vi "donut_fitting(subVI).vi"(5 "Edge Options":T1={"Edge Polarity"=0, "Kernel Size"=3, "Width"=3, "Minimum Edge Strength"=10.0, "Interpolation Type"=enum."Bilinear Fixed", "Data Processing Method"=enum."Average"} {"Edge Polarity" items=["All Edges", "Rising Edges", "Falling Edges"]; "Minimum Edge Strength" format="%.2f"; "Width" step=2; "Kernel Size" step=2}, 7 "Scan Direction":u16(ring) items=["Outside To Inside", "Inside To Outside"], 8 "error in (no error)":errorcluster, 9 "Step Size":dbl=5.0 format="%#_13g", 10 "image dest":T3, 11 "Image in":T3) -> (0 "error out":errorcluster, 3 "Image Out":T3)   [LabVIEW 2020]
uses:
  <vilib>/vision/Image Controls.llb/IMAQ Image.ctl
  <vilib>/vision/Measure.llb/Edge Options.ctl
  <vilib>/vision/Measure.llb/Edge Polarity.ctl
  <vilib>/vision/NI_Vision_Development_Module.lvlib
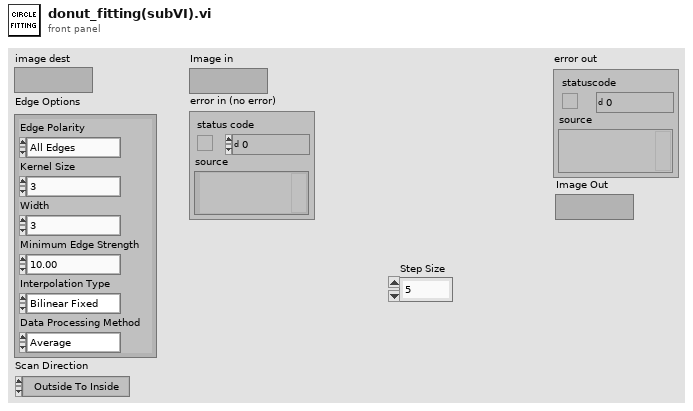
[diagram p1: front panel]
types:
  T1 = typedef "Edge Options.ctl" = cluster{"Edge Polarity":T2, "Kernel Size":u32, "Width":u32, "Minimum Edge Strength":sgl, "Interpolation Type":enum32{"Zero Order", "Bilinear", "Quadratic", "Cubic", "Bilinear Fixed"}, "Data Processing Method":enum32{"Average", "Median"}}
  T2 = typedef "Edge Polarity.ctl" = u32
  T3 = typedef "IMAQ Image.ctl" = refnum<image>
  T4 = typedef "ROI Descriptor" = cluster{"Global Rectangle":i32[], "Contours":cluster{"ID":enum32{"External", "Internal"}, "Type":u32, "Coordinates":i32[]}[]}
  T5 = typedef "Edge New.ctl" = cluster{"Location (Pixel)":cluster{"X":sgl, "Y":sgl}, "Location (Real-World)":cluster{"X":sgl, "Y":sgl}, "Distance (Pixel)":dbl, "Distance (Real-World)":dbl, "Strength":dbl, "Noise":dbl, "Rising?":bool}
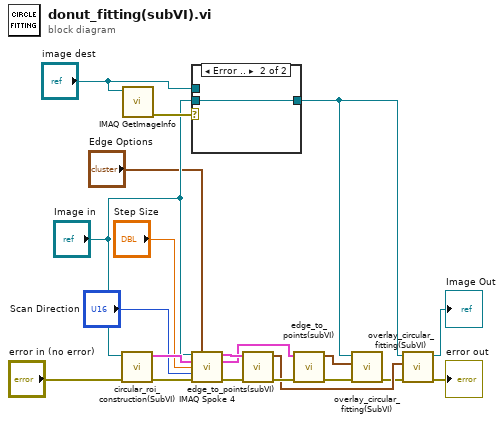
[diagram p0: block diagram]
diagram:
  n1 = call "circular_roi_construction(SubVI).vi"("error in (no error)"="error in (no error)", "image in"="Image in") -> ("error out"=w19:errorcluster, "ROI Descriptor"=w20:T4)  [unwired: 8 in]
  n2 = call "IMAQ GetImageInfo"("Image"="image dest") -> ("error out"=w7:errorcluster)  [unwired: 3 in, 7 out]
  n3 = case shown="Error .." w7 {
    tunnel: "image dest" -> [w21 _]
    tunnel: [w21 w22] -> w5
    tunnel: "Image in" -> [_ w22]
    frame No Error {
    }
    frame Error {
    }
  }
  n4 = call "IMAQ Spoke 4"("Image"="Image in", "Edge Options"="Edge Options", "ROI Descriptor"=w20, "Step Size"="Step Size", "Scan Direction"="Scan Direction", "error in (no error)"=w19) -> ("First Edges"=w17:T5[], "Last Edges"=w16:T5[], "error out"=w15:errorcluster)  [unwired: 6 in, 1 out]
  n5 = call "edge_to_points(subVI).vi"("error in (no error)"=w15, "First Edges"=w17) -> ("error out"=w14:errorcluster, "points (pixel)"=w12:cluster{"X":sgl, "Y":sgl}[])  [unwired: 7 in, 1 out]
  n6 = call "edge_to_points(subVI).vi"("error in (no error)"=w14, "First Edges"=w16) -> ("error out"=w9:errorcluster, "points (pixel)"=w13:cluster{"X":sgl, "Y":sgl}[])  [unwired: 7 in, 1 out]
  n7 = call "overlay_circular_fitting(SubVI).vi"("error in (no error)"=w9, "points (pixel)"=w13, "image dest"=w5) -> ("error out"=w11:errorcluster)  [unwired: 6 in, 2 out]
  n8 = call "overlay_circular_fitting(SubVI).vi"("error in (no error)"=w11, "points (pixel)"=w12, "image dest"=w5) -> ("error out"=→"error out":errorcluster, "Image Out"=→"Image Out":T3)  [unwired: 6 in, 1 out]
